vi "Read SequenceValues.vi"(8 "error in (no error)":errorcluster, 11 "VariableManager in":refnum<class "VariableManager.lvclass">) -> (0 "error out":errorcluster, 2 "SequenceValues":refnum<class "VariableValue.lvclass">[][](array[class]), 3 "VariableManager out":refnum<class "VariableManager.lvclass">)   [LabVIEW 2013, in "VariableManager.lvclass"]
uses:
  VariableManager.lvclass
  VariableValue/VariableValue.lvclass
  VariableManager.lvclass/VariableManager.ctl
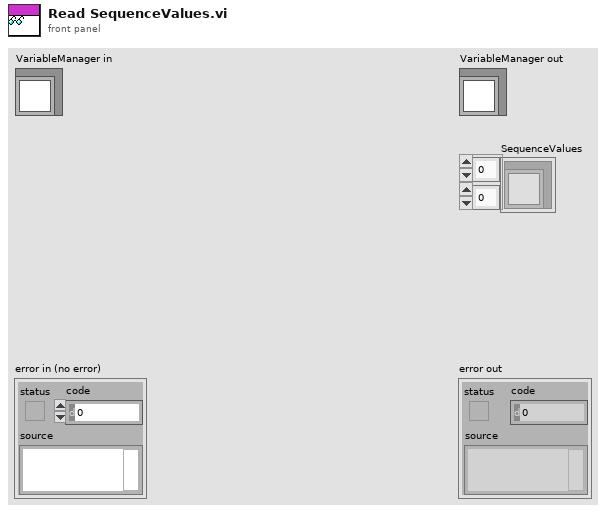
[diagram p1: front panel]
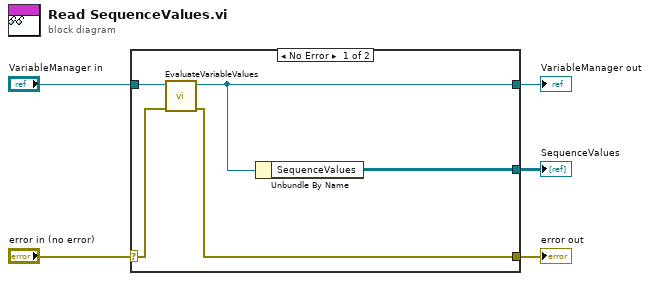
[diagram p0: block diagram]
diagram:
  n1 = case shown="No Error" "error in (no error)" {
    selector: "error in (no error)" -> [w7 w11]
    tunnel: [w6 w11] -> w4
    tunnel: [w8 w12] -> w2
    tunnel: "VariableManager in" -> [w9 w12]
    tunnel: [w10 _] -> w1
    frame No Error {
      n2 = call-dynamic "EvaluateVariableValues.vi"("error in (no error)"=w7, "VariableManager in"=w9) -> ("error out"=w6:errorcluster, "VariableManager out"=w8:refnum<class "VariableManager.lvclass">)  [unwired: 8 in]
      n3 = Unbundle By Name(w8) -> ("SequenceValues"=w10:refnum<class "VariableValue.lvclass">[][])
    }
    frame Error {
    }
  }
  "error out" <- w4
  "VariableManager out" <- w2
  "SequenceValues" <- w1
